vi "Write Trigger Settings.vi"(8 "error in":errorcluster, 10 "Trigger Settings":T1={"Edge:"=0, "Level"=0.0, "Source"=0, "trigger coupling"=1, "Holdoff"=0.0, "Delay"=0.0, "Trigger Modifier"=enum."Auto Trigger", "Trigger Type"=enum."Digital"} {"Delay" format="%_6g"; "Holdoff" format="%_6g"; "trigger coupling" items=["AC", "DC", "HF Reject", "LF Reject", "AC Plus HF Reject"]; "Source" items=["Channel_1", "Channel_2", "Channel_3", "Channel_4", "Channel_5", "Channel_6", "Channel_7", "Channel_8"]; "Level" format="%_6g"; "Edge:" items=["Rising Edge", "Falling Edge"]}, 11 "Oscilloscope in":refnum<class "Oscilloscope.lvclass">) -> (0 "error out":errorcluster, 3 "Oscilloscope out":refnum<class "Oscilloscope.lvclass">)   [LabVIEW 2019, in "Oscilloscope.lvlib" / "Oscilloscope.lvclass"]
uses:
  Oscilloscope.lvclass
  Custom Controls/Trigger Settings.ctl
  Custom Controls/Edge Select.ctl
  Custom Controls/Channel List.ctl
  Custom Controls/Trigger Coupling.ctl
  Custom Controls/Trigger Modifier.ctl
  Custom Controls/Trigger Type.ctl
  Oscilloscope.lvclass/Oscilloscope.ctl
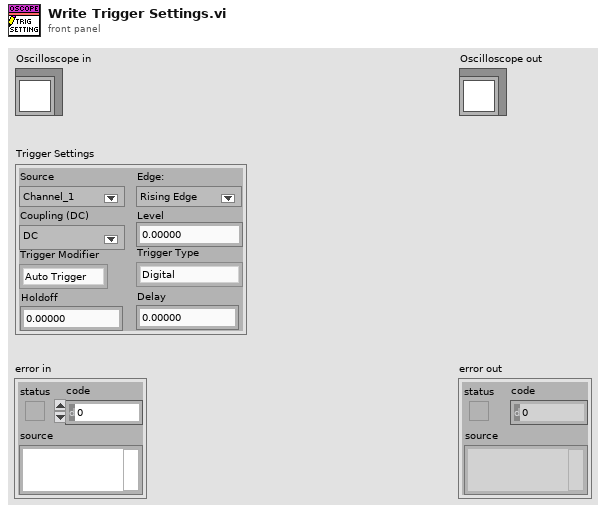
[diagram p1: front panel]
types:
  T1 = typedef "Oscilloscope.lvlib/Oscilloscope.lvclass/Trigger Settings.ctl" = cluster{"Edge:":T2, "Level":dbl, "Source":T3, "trigger coupling":T4, "Holdoff":dbl, "Delay":dbl, "Trigger Modifier":T5, "Trigger Type":T6}
  T2 = typedef "Oscilloscope.lvlib/Oscilloscope.lvclass/Edge Select.ctl" = u16
  T3 = typedef "Oscilloscope.lvlib/Oscilloscope.lvclass/Channel List.ctl" = u16
  T4 = typedef "Oscilloscope.lvlib/Oscilloscope.lvclass/Trigger Coupling.ctl" = u16
  T5 = typedef "Oscilloscope.lvlib/Oscilloscope.lvclass/Trigger Modifier.ctl" = enum16{"Invalid_Setting", "None", "Auto Trigger"}
  T6 = typedef "Oscilloscope.lvlib/Oscilloscope.lvclass/Trigger Type.ctl" = enum16{"Immediate", "Analog Edge", "Digital", "Window", "Hysteresis"}
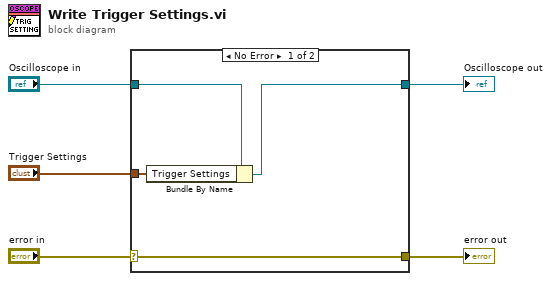
[diagram p0: block diagram]
diagram:
  n1 = case shown="No Error" "error in" {
    selector: "error in" -> [w6 w10]
    tunnel: [w6 w10] -> w2
    tunnel: [w7 w11] -> w1
    tunnel: "Oscilloscope in" -> [w9 w11]
    tunnel: "Trigger Settings" -> [w8 _]
    frame No Error {
      n2 = Bundle By Name(cluster=w9, "Trigger Settings"=w8) -> (w7:refnum<class "Oscilloscope.lvclass">)
    }
    frame Error {
    }
  }
  "error out" <- w2
  "Oscilloscope out" <- w1
